vi "Preston_shear_stress.vi"(4 "Head correction (mmH2O)":dbl, 5 "Calib. consts":dbl[](array[numeric]) format="%#_12g", 6 "Diam. (mm)":dbl, 7 "Temp (C)":dbl, 8 "Static gauge head mm H2O":dbl, 9 "Atmos. pressure (mbars)":dbl, 10 "Pressure transducer voltages":dbl[](array[numeric])) -> (3 "Mean shear stress (Pa)":dbl)   [LabVIEW 2010]
uses:
  <vilib>/Analysis/NI_AALBase.lvlib
panel:
  # "Use this if you connected the wrong static pressure to the manometer and know what the error is."
  # "If tau is NaN, then you have used the Preston tube outside its applicable range!"
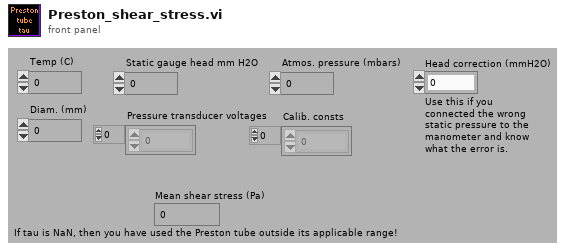
[diagram p1: front panel]
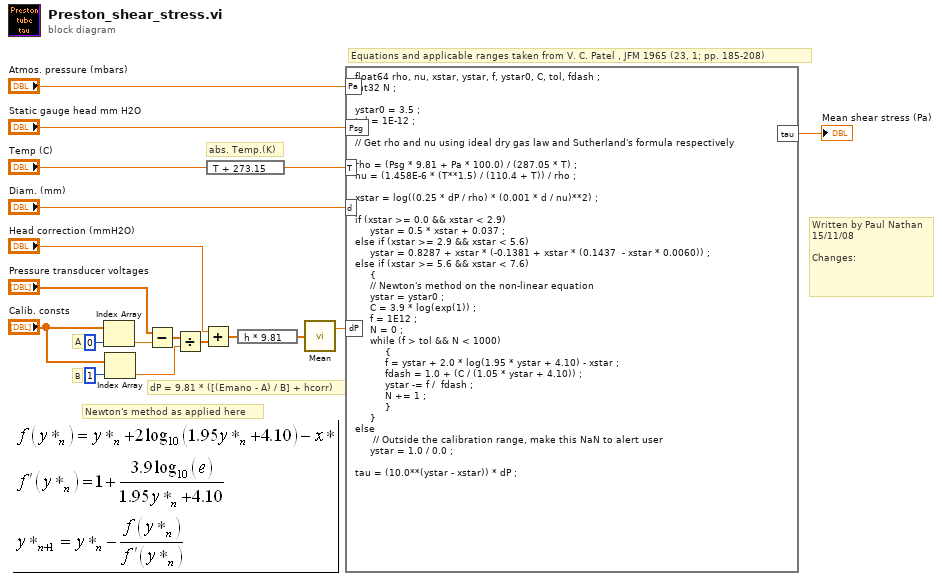
[diagram p0: block diagram]
diagram:
  # "Written by Paul Nathan\n15/11/08\n\nChanges:"
  # "Newton's method as applied here"
  # "abs. Temp.(K)"
  # "Equations and applicable ranges taken from V. C. Patel , JFM 1965 (23, 1; pp. 185-208)"
  # "B"
  # "A"
  # "dP = 9.81 * ([(Emano - A) / B] + hcorr)"
  n1 = Index Array(array="Calib. consts", index=0) -> (element=w12:dbl)
  n2 = Index Array(array="Calib. consts", index=1) -> (element=w10:dbl)
  n3 = Subtract(x="Pressure transducer voltages", y=w12) -> (x-y=w11:dbl[])
  n4 = Divide(x=w11, y=w10) -> (x/y=w2:dbl[])
  n5 = Add(x="Head correction (mmH2O)", y=w2) -> (x+y=w3:dbl[])
  n6 = expression code="T + 273.15"("Temp (C)") -> (w4:dbl)
  n7 = expression code="h * 9.81"(w3) -> (w9:dbl[])
  n8 = call <vilib>:"Mean.vi"("X"=w9) -> ("mean"=w7:dbl)  [unwired: 1 out]
  n9 = formula code="float64 rho, nu, xstar, ystar, f, ystar0, C, tol, fdash ;\nint32 N ;\n\nystar0 = 3.5 ;\ntol = 1E-12 ;\n\n// Get rho and nu using ideal dry gas law and Sutherland's formula respectively\n\nrho = (Psg * 9.81 + Pa * 100.0) / (287.05 * T) ;\nnu = (1.458E-6 * (T**1.5) / (110.4 + T)) / rho ;\n\nxstar = log((0.25 * dP / rho) * (0.001 * d / nu)**2) ;\n\nif (xstar >= 0.0 && xstar < 2.9)\n     ystar = 0.5 * xstar + 0.037 ;\nelse if (xstar >= 2.9 && xstar < 5.6)\n     ystar = 0.8287 + xstar * (-0.1381 + xstar * (0.1437  - xstar * 0.0060)) ;\nelse if (xstar >= 5.6 && xstar < 7.6) \n     {\n     // Newton's method on the non-linear equation\n     ystar = ystar0 ;\n     C = 3.9 * log(exp(1)) ;\n     f = 1E12 ;\n     N = 0 ;\n     while (f > tol && N < 1000)\n          {\n          f = ystar + 2.0 * log(1.95 * ystar + 4.10) - xstar ;\n          fdash = 1.0 + (C / (1.05 * ystar + 4.10)) ;\n          ystar -= f /  fdash ;\n          N += 1 ;\n          }\n     }\nelse\n      // Outside the calibration range, make this NaN to alert user\n     ystar = 1.0 / 0.0 ;\n\ntau = (10.0**(ystar - xstar)) * dP ;"("T"=w4, "Psg"="Static gauge head mm H2O", "Pa"="Atmos. pressure (mbars)", "dP"=w7, "d"="Diam. (mm)") -> ("tau"=→"Mean shear stress (Pa)":dbl)
